vi "ReadHardwareConfigure.vi"(8 "error in (no error)":errorcluster, 11 "Hardware Resources in":T1) -> (0 "error out":errorcluster, 2 "Output Registers":i32[](array[numeric]), 3 "Hardware Resources out":T1)   [LabVIEW 2016]
uses:
  Hardware Configuration.ctl
  <vilib>/NI Modbus.llb/MB Serial Master Query Read Holding Registers (poly).vi
  Acquisition.lvlib
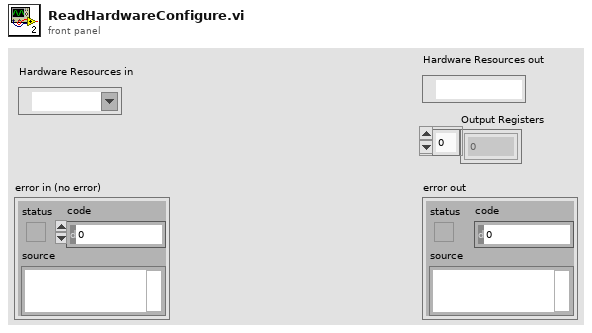
[diagram p1: front panel]
types:
  T1 = typedef "Acquisition.lvlib/Hardware Configuration.ctl" = refnum<visa-resource-name>
  T2 = cluster{"Mode":enum16{"RTU", "ASCII"}, "Slave Address":u8}
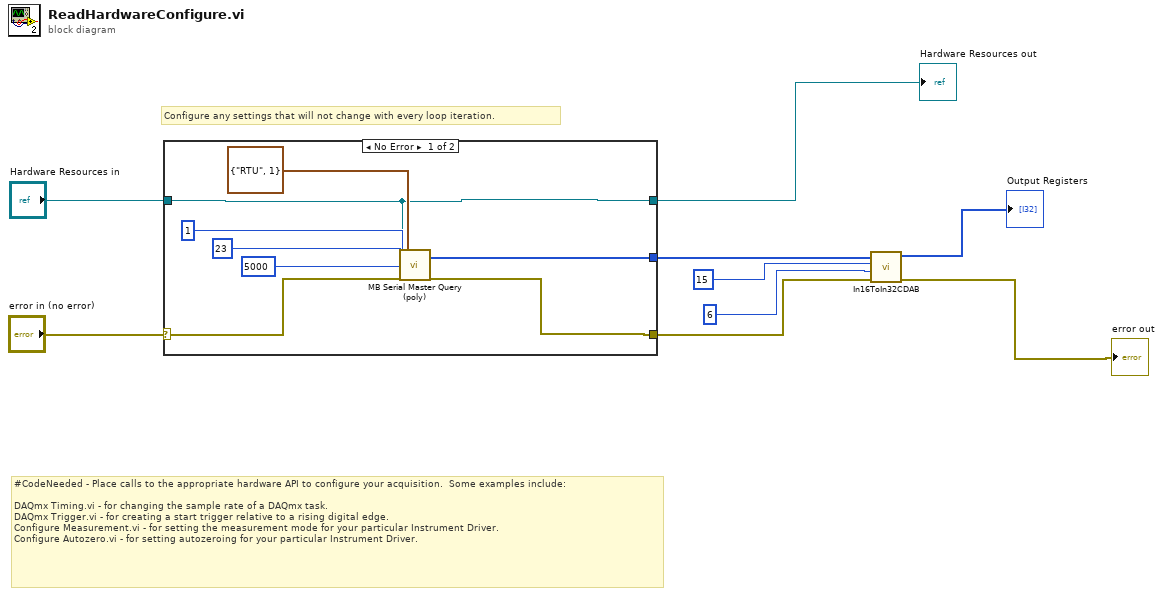
[diagram p0: block diagram]
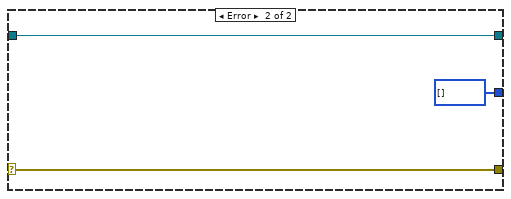
[diagram p2: hidden frame]
diagram:
  # "Configure any settings that will not change with every loop iteration."
  # "#CodeNeeded - Place calls to the appropriate hardware API to configure your acquisition.  Some examples include:\n\nDAQmx Timing.vi - for changing the sample rate of a DAQmx task.\nDAQmx Trigger.vi - for creating a start trigger relative to a rising digital edge.\nConfigure Measurement.vi - for setting the measurement mode for your particular Instrument Driver.\nConfigure Autozero.vi - for setting autozeroing for your particular Instrument Driver."
  n1 = case shown="No Error" "error in (no error)" {
    selector: "error in (no error)" -> [w16 w19]
    tunnel: [w17 w19] -> w5
    tunnel: "Hardware Resources in" -> [w10 w20]
    tunnel: [w10 w20] -> w7
    tunnel: [w11 u16[] [] ("Input Registers")] -> w6
    frame No Error {
      n2 = call-poly <vilib>:"MB Serial Master Query (poly).vi"("VISA resource name"=w10, "Starting Address"=u16 1, "Quantity"=u16 23, "Timeout"=u32 5000, "error in"=w16, "Serial Parameters"=T2 {"Mode"=enum."RTU", "Slave Address"=1}) -> ("Holding Registers"=w11:u16[], "error out"=w17:errorcluster)  [unwired: 10 in, 2 out]
    }
    frame Error {
    }
  }
  "Hardware Resources out" <- w7
  n3 = call "In16ToIn32CDAB.vi"("error in (no error)"=w5, "length"=6, "index"=15, "Input Registers"=w6) -> ("error out"=→"error out":errorcluster, "Output Registers"=→"Output Registers":i32[])  [unwired: 6 in]
